vi "PM-A-myDAQ-init.vi"(8 "error in":errorcluster) -> (0 "error out":errorcluster, 3 "Refnum out":refnum<k21>)   [LabVIEW 2018]
uses:
  <vilib>/DAQmx/create/channels.llb/DAQmx Create Channel (AI-Voltage-Basic).vi
  <vilib>/DAQmx/configure/timing.llb/DAQmx Timing (Sample Clock).vi
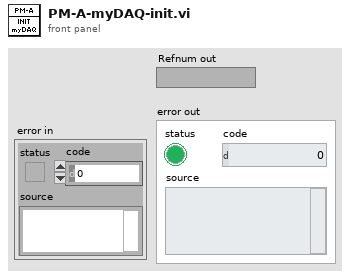
[diagram p1: front panel]
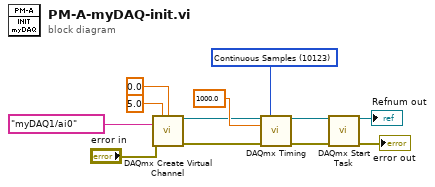
[diagram p0: block diagram]
diagram:
  w5 = 10123 items=["Finite Samples"=10178, "Continuous Samples"=10123, "Hardware Timed Single Point"=12522] ("sample mode")
  n1 = call-poly <vilib>:"DAQmx Create Virtual Channel.vi"("maximum value"=5.0, "minimum value"=0.0, "physical channels"=tag "myDAQ1/ai0", "error in"="error in") -> ("task out"=w2:refnum<k21>, "error out"=w3:errorcluster)  [unwired: 10 in]
  n2 = call-poly <vilib>:"DAQmx Timing.vi"("task/channels in"=w2, "sample mode"=w5, "rate"=1000.0, "error in"=w3) -> ("task out"=w10:refnum<k21>, "error out"=w7:errorcluster)  [unwired: 10 in]
  n3 = call <vilib>:"DAQmx Start Task.vi"("task/channels in"=w10, "error in"=w7) -> ("task out"=→"Refnum out":refnum<k21>, "error out"=→"error out":errorcluster)  [unwired: 12 in]
